vi "WRITE.vi"(9 "Value":i8, 11 "Python in":string) -> (3 "Python out":string)   [LabVIEW 2016]
panel:
  out "bytes added":u8[](array[numeric])=[64, 35, 0] format="%.0x"
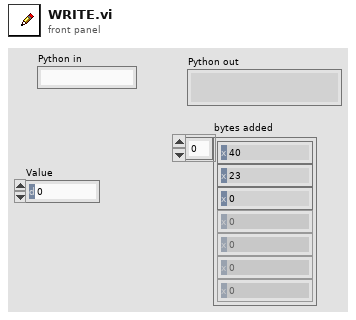
[diagram p1: front panel]
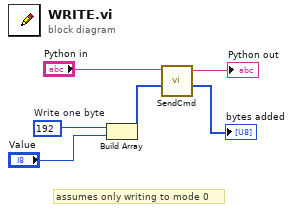
[diagram p0: block diagram]
diagram:
  w2 = u8 192  # Write one byte
  # "assumes only writing to mode 0"
  n1 = Build Array(w2, "Value") -> (w3:u8[])
  n2 = call "SendCmd.vi"("Array In"=w3, "Python in"="Python in") -> ("Array Sent"=→"bytes added":u8[], "Python out"=→"Python out":string)  [unwired: 8 in]
